vi "Shutdown.vi"(8 "error in (no error)":errorcluster, 11 "View in":refnum<class "View.lvclass">) -> (0 "error out":errorcluster, 3 "View out":refnum<class "View.lvclass">)   [LabVIEW 2020, in "Page1.lvlib" / "View.lvclass"]
uses:
  View.lvclass
  View.lvclass/View.ctl
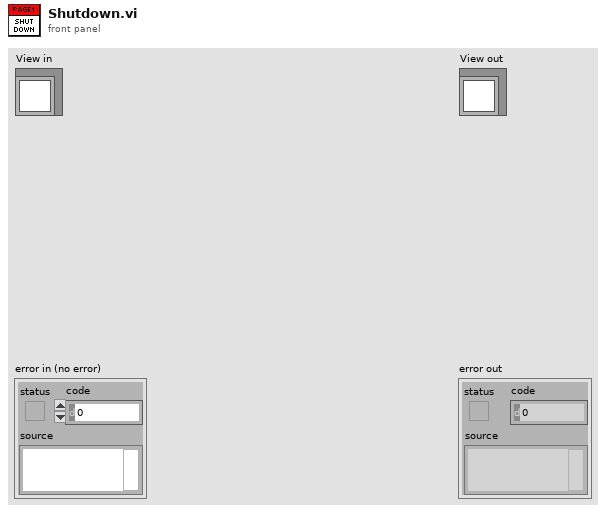
[diagram p1: front panel]
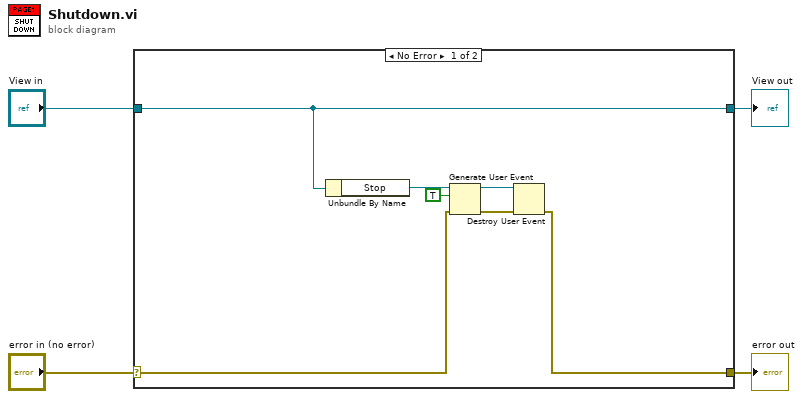
[diagram p0: block diagram]
diagram:
  n1 = case shown="No Error" "error in (no error)" {
    selector: "error in (no error)" -> [w8 w13]
    tunnel: [w6 w13] -> w3
    tunnel: "View in" -> [w5 w12]
    tunnel: [w5 w12] -> w1
    frame No Error {
      n2 = Unbundle By Name(w5) -> ("Stop"=w11:refnum<user-event>)
      n3 = Generate User Event(user event=w11, event data cluster=TRUE ("event data"), error in=w8) -> (user event out=w10:refnum<user-event>, error out=w7:errorcluster)  [unwired: 1 in]
      n4 = Destroy User Event(user event=w10, error in=w7) -> (error out=w6:errorcluster)
    }
    frame Error {
    }
  }
  "error out" <- w3
  "View out" <- w1
